vi "integral.vi"(8 "Reset":bool, 10 "Starting value":dbl, 11 "x":dbl) -> (3 "Integral x":dbl)   [LabVIEW 2017]
doc: "Takes the integral of x with respect to time. Uses the rectangle method of integration"
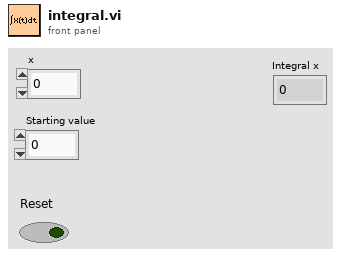
[diagram p1: front panel]
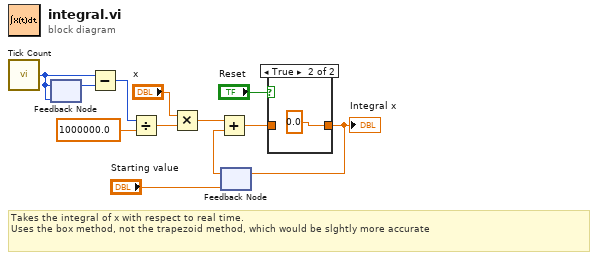
[diagram p0: block diagram]
diagram:
  # "Takes the integral of x with respect to real time.\nUses the box method, not the trapezoid method, which would be slghtly more accurate"
  n1 = call "Tick Count"() -> ("Tick Count(uSec)"=w1:u32)
  n2 = feedback #1(w1) -> (w11:u32)
  n3 = feedback-in #1(w1) -> ()
  n4 = Subtract(x=w1, y=w11) -> (x-y=w7:u32)
  n5 = Divide(x=w7, y=1000000.0) -> (x/y=w5:dbl)
  n6 = Multiply(x="x", y=w5) -> (x*y=w9:dbl)
  n7 = feedback #2("Starting value") -> (w8:dbl)
  n8 = Add(x=w9, y=w8) -> (x+y=w2:dbl)
  n9 = case shown="True" "Reset" {
    tunnel: [w13 0.0] -> w3
    tunnel: w2 -> [w13 _]
    frame False {
    }
    frame True {
    }
  }
  "Integral x" <- w3
  n10 = feedback-in #2(w3) -> ()
